vi "Create.vi"(5 "ErrorMessageContains In":refnum<class "ErrorMessageContains.lvclass">, 8 "error in (no error)":errorcluster, 10 "Expected":string) -> (0 "error out":errorcluster, 3 "ErrorMessageContains":refnum<class "ErrorMessageContains.lvclass">)   [LabVIEW 2019, in "Constraint.lvlib" / "ErrorMessageContains.lvclass"]
uses:
  ErrorMessageContains.lvclass
  ErrorMessageContains.lvclass/ErrorMessageContains.ctl
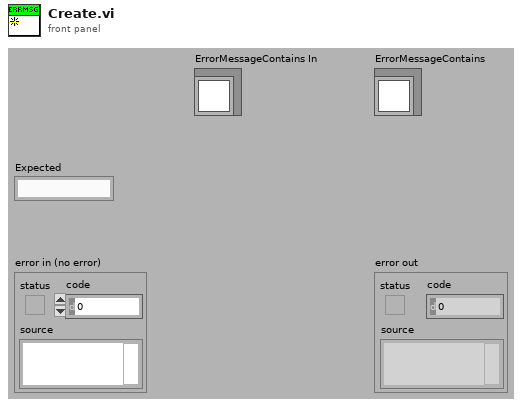
[diagram p1: front panel]
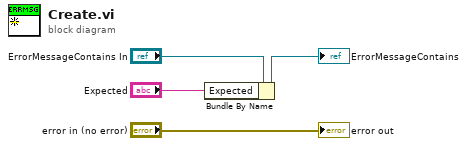
[diagram p0: block diagram]
diagram:
  n1 = Bundle By Name(cluster="ErrorMessageContains In", "Expected"="Expected") -> (→"ErrorMessageContains":refnum<class "ErrorMessageContains.lvclass">)
  "error out" <- "error in (no error)"
